vi "Acq Fetch Trigger Delay.vi"(0 "session in":refnum<class "Digitizer Control.lvclass">, 2 "records to read":u32, 5 "error in (no error)":errorcluster, 7 "timeout (ms)":i32=5000) -> (14 "session out":refnum<class "Digitizer Control.lvclass">, 15 "trigger delay (s)":dbl[](array[numeric]), 16 "samples to ignore":i32[](array[numeric]), 18 "records remaining":u32, 19 "error out":errorcluster)   [LabVIEW 2021, in "Digitizer Control.lvclass"]
doc: "Fetches the recorded trigger synchronization delays. TClk synchronized acquisitions have an inherent trigger response latency that is between 1-2 TClk periods. The latency can be compensated by acquiring additional pre-trigger samples and keeping only latency worth of the additional pre-trigger samples. When using TClk synchronization, use the <B>Acq Configure Pretrigger Period.vi</B> on all devices to enable the acquisition of the additional pre-trigger samples, and enable the recording of the delay between the device receiving a trigger and starting the acquisition on the master device (using the <B>trigger delay tracking enable</B> input of the <B>Acq Configure Transfer.vi</B>). When fetching a record, use this VI on the master device to fetch the recorded delay value and the number of samples to remove from the beginning of the record to align the record with the trigger.\n\nInputs:\n\n<B>session in</B>: The device session.\n\n<B>records to read</B>: The number of recorded trigger delays to fetch.\n\n<B>timeout</B>: The maximum amount of time, in milliseconds, this VI is allowed to wait for the recorded trigger delays to become available.\n\nOutputs:\n\n<B>session out</B>: The device session passed on the <B>session in</B> input.\n\n<B>trigger delay (s)</B>: Array of the fetched trigger delays, scaled to seconds.\n\n<B>samples to ignore</B>: Array of the number of samples to remove from the beginning of the corresponding records.\n\n<B>records remaining</B>: The number of additional trigger delays remaining in the host DMA buffer that are available for reading."
uses:
  Digitizer Control.lvclass
  Digitizer Control.lvclass/Digitizer Control.ctl
  <vilib>/Utility/error.llb/Error Cluster From Error Code.vi
  <vilib>/rvi/errors/niLvFpgaAdjustHostInterfaceError.vi
  <vilib>/ErrorRing/Error Ring.xnode
  <vilib>/rvi/interface/nirviMethod/nirviMethod.xnode
  <vilib>/FPGAPlugInAG/Dynamic/niLvFpga_ReadFifo_Dynamic.vi
  <vilib>/rvi/errors/niLvFpgaMergeErrorWithErrorCode.vi
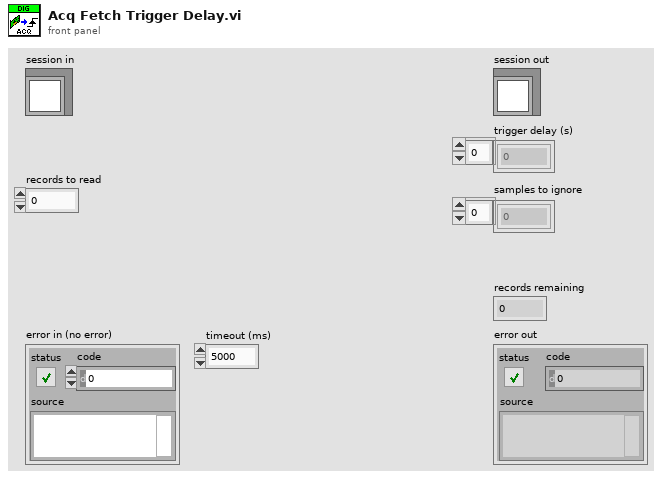
[diagram p1: front panel]
types:
  T1 = typedef "Digitizer Control.lvclass/Acq Session Data.ctl" = cluster{"ADC sampling rate":dbl, "SCTL rate":dbl, "DMA element size (bits)":i32, "sample size (bits)":i32[], "DMA/memory interface width (DMA elements)":i32, "transfer size (bits)":i32[], "stream instance":i32[], "trigger instance":u32, "group delay (s)":dbl, "data delay (s)":dbl, "target delay (s)":dbl, "trigger tracking enabled":bool, "channel configured":bool, "enabled channels":bool[], "transfer configured":bool, "dsp bypass":bool, "fractional decimator input rate":dbl, "fractional decimator output rate":dbl, "sample scale factor":dbl[], "memory size":u64[], "FIFO size":u64}
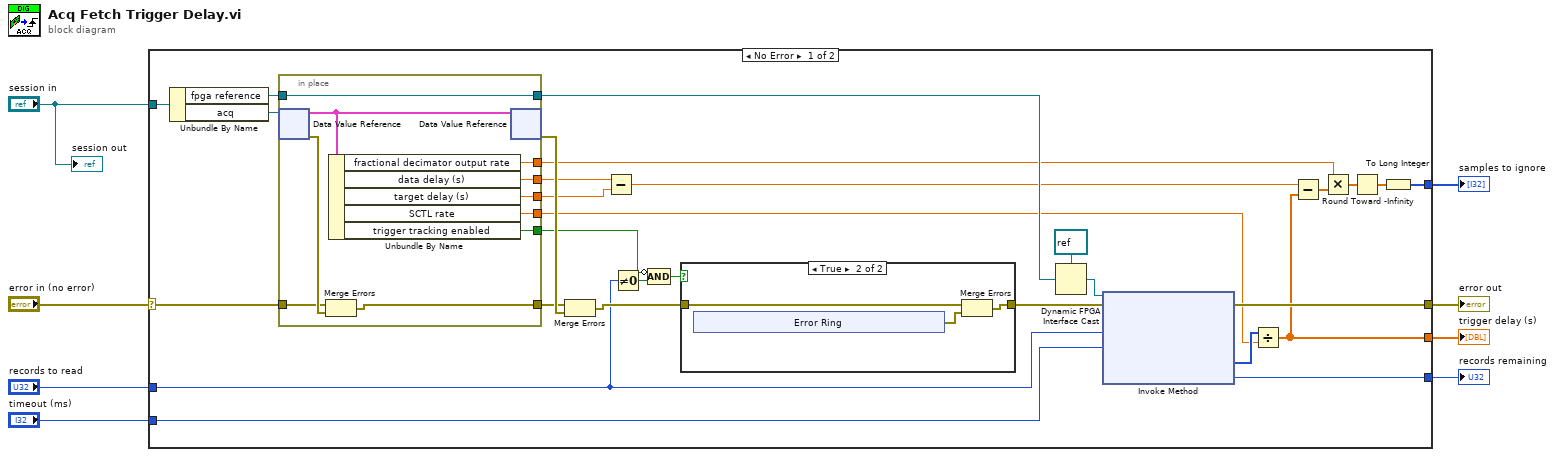
[diagram p0: block diagram]
diagram:
  n1 = case shown="No Error" "error in (no error)" {
    selector: "error in (no error)" -> [w33 w57]
    tunnel: "records to read" -> [w27 _]
    tunnel: [w19 w57] -> w6
    tunnel: "timeout (ms)" -> [w34 _]
    tunnel: [w15 _] -> w4
    tunnel: "session in" -> [w30 _]
    tunnel: [w31 _] -> w3
    tunnel: [w9 _] -> w1
    frame No Error {
      n2 = Unbundle By Name(w30) -> ("fpga reference"=w28:refnum<k20>, "acq"=w29:refnum<data-value>)
      n3 = in-place {
        in-place-border: w33 -> [w55]
        in-place-border: [w53] -> w24
        in-place-border: [w52] -> w32
        in-place-border: w28 -> [w51]
        in-place-border: [w51] -> w37
        in-place-border: [w50] -> w18
        in-place-border: [w49] -> w17
        in-place-border: [w48] -> w16
        in-place-border: [w47] -> w12
        n4 = in-place-dvr #1(w29) -> (w54:T1, w56:errorcluster)
        n5 = Merge Errors(w55, w56) -> (w52:errorcluster)
        n6 = Unbundle By Name(w54) -> ("fractional decimator output rate"=w47:dbl, "data delay (s)"=w49:dbl, "target delay (s)"=w48:dbl, "SCTL rate"=w50:dbl, "trigger tracking enabled"=w53:bool)
        n7 = in-place-dvr #1(w54) -> (w35:errorcluster)  [unwired: 1 out]
      }
      n8 = Merge Errors(w32, w35) -> (w36:errorcluster)
      n9 = Subtract(x=w17, y=w16) -> (x-y=w14:dbl)
      n10 = Not Equal To 0?(x=w27) -> (x != 0?=w26:bool)
      n11 = Compound Arithmetic op=AND(invert w24, w26) -> (w25:bool)
      n12 = case shown="True" w25 {
        tunnel: w36 -> [w38 w41]
        tunnel: [w38 w39] -> w23
        frame False {
        }
        frame True {
          n13 = xnode "Error Ring"() -> ("error out"=w40:errorcluster)
          n14 = Merge Errors(w41, w40) -> (w39:errorcluster)
        }
      }
      n15 = Dynamic FPGA Interface Cast(Session In=refnum<k20> refnum ("Type"), Type=w37) -> (Session Out=w20:refnum<k20>)
      n16 = xnode "Invoke Method"("FPGA VI Reference In"=w20, "error in"=w23, "Number of Elements"=w27, "Timeout (ms)"=w34) -> ("error out"=w19:errorcluster, "Data"=w21:u32[], "Elements Remaining"=w31:u32)  [unwired: 1 out]
      n17 = Divide(x=w21, y=w18) -> (x/y=w15:dbl[])
      n18 = Subtract(x=w14, y=w15) -> (x-y=w13:dbl[])
      n19 = Multiply(x=w12, y=w13) -> (x*y=w11:dbl[])
      n20 = Round Toward -Infinity(1:w11) -> (0:w10:dbl[])
      n21 = To Long Integer(number=w10) -> (32bit integer=w9:i32[])
    }
    frame Error {
    }
  }
  "error out" <- w6
  "trigger delay (s)" <- w4
  "records remaining" <- w3
  "samples to ignore" <- w1
  "session out" <- "session in"
